vi "EssUI.vi"() -> ()   [LabVIEW 2018]
panel:
  in  "Mint 7":string
  in  "Maxt 6":string
  in  "Status 8":string
  in  "Minv 5":string
  in  "Maxv 4":string
  in  "SOC 1":string
  in  "Curr 3":string
  in  "Sumv 2":string
  in  "Mint 5":string
  in  "Maxt 5":string
  in  "Status 5":string
  in  "Minv 5":string
  in  "Maxv 5":string
  in  "SOC 5":string
  in  "Curr 5":string
  in  "Sumv 5":string
  in  "Mint 4":string
  in  "Maxt 4":string
  in  "Status 4":string
  in  "Minv 4":string
  in  "Maxv 4":string
  in  "SOC 4":string
  in  "Curr 4":string
  in  "Sumv 4":string
  in  "Mint 3":string
  in  "Maxt 3":string
  in  "Status 3":string
  in  "Minv 3":string
  in  "Maxv 3":string
  in  "SOC 3":string
  in  "Curr 3":string
  in  "Sumv 3":string
  in  "Mint 2":string
  in  "Maxt 2":string
  in  "Status 2":string
  in  "Minv 2":string
  in  "Maxv 2":string
  in  "SOC 2":string
  in  "Curr 2":string
  in  "Sumv 2":string
  in  "Status":string
  in  "SOC":string
  in  "Curr":string
  in  "Sumv":string
  in  "Boolean 4":bool
  in  "Boolean 3":bool
  in  "Boolean 2":bool
  in  "Boolean":bool
  # "BMS Monitor"
  # "总信息"
  # "电池组2"
  # "电池组3"
  # "电池组1"
  # "电池组4"
  # "电池组5"
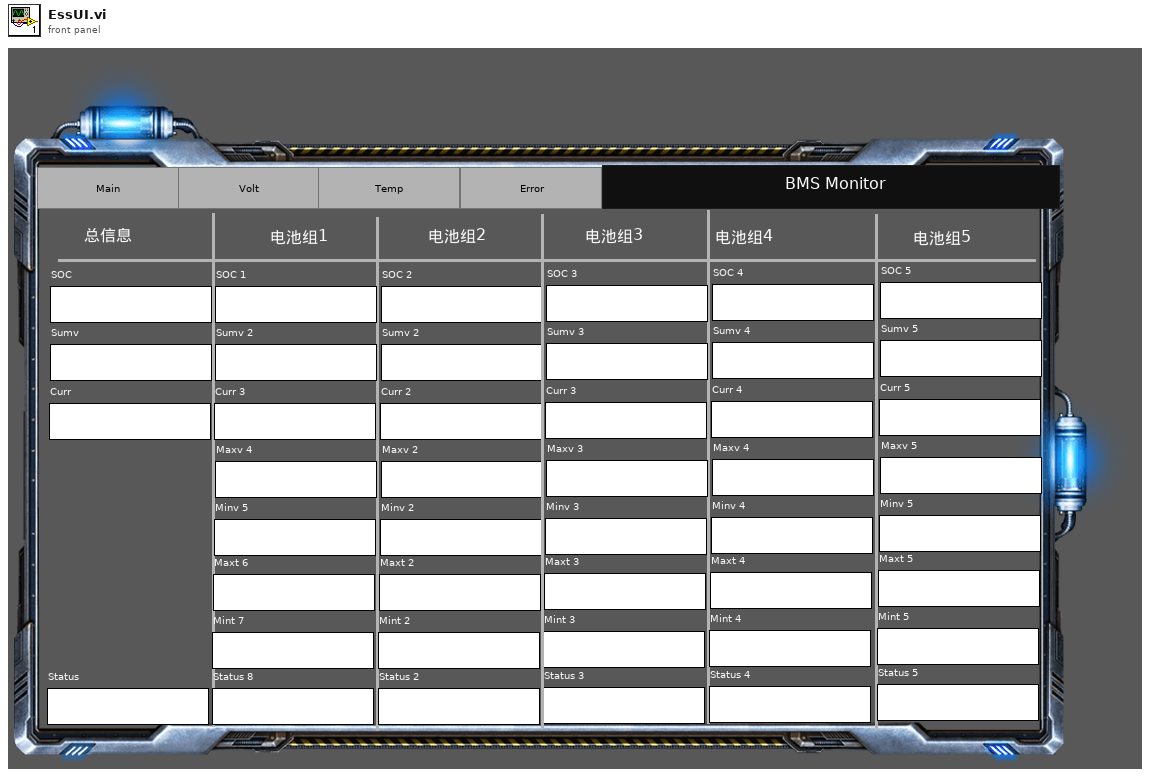
[diagram p1: front panel]
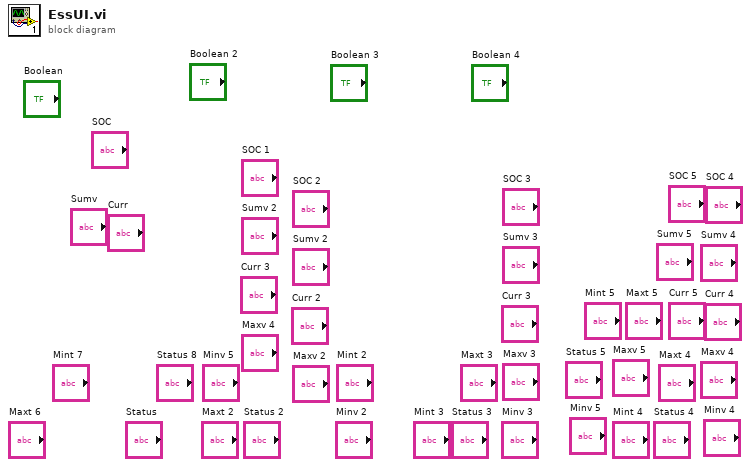
[diagram p0: block diagram]
diagram:
